vi "AlazarSetClockSwitchOver.vi"(3 "error in (no error)":errorcluster, 4 "DummyClockOnTime_ns":u32, 5 "Mode":u32(ring) items=["Disable", "Enable"], 6 "Handle":u64) -> (0 "error out":errorcluster, 1 "Return Code":u32, 2 "Handle":u64)   [LabVIEW 2009]
doc: "Configure the dummy clock.\n\nWhen the \"dummy clock\" option enabled, the digitizer uses an internally generated clock signal to drive its ADCs for a specified amount of time after the end of each record. At the end of the dummy clock on time, the digitizer switches back to using the external clock signal to clock the ADCs.\n\nScanning applications that generate an unusable external clock signal during horizontal retrace periods at the end of each scan line should consider enabling the \"dummy clock\" option."
uses:
  ATSApi.dll
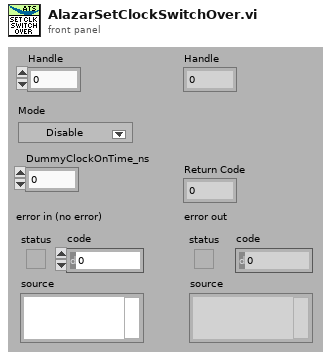
[diagram p1: front panel]
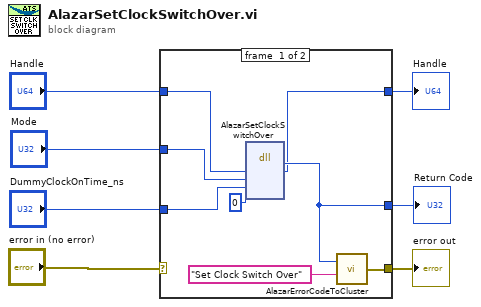
[diagram p0: block diagram]
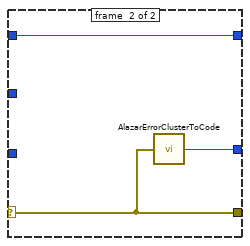
[diagram p2: hidden frame]
diagram:
  n1 = case shown="No Error" "error in (no error)" {
    selector: "error in (no error)" -> [_ w18]
    tunnel: [w12 w18] -> w6
    tunnel: [w14 w17] -> w5
    tunnel: "Handle" -> [w15 w16]
    tunnel: [w11 w16] -> w3
    tunnel: "Mode" -> [w10 _]
    tunnel: "DummyClockOnTime_ns" -> [w9 _]
    frame #0 {
      n2 = dll-call lib="ATSApi.dll" fn="AlazarSetClockSwitchOver"("handle"=w15, "mode"=w10, "dummyClockOnTime_ns"=w9, "reserved"=u32 0) -> ("return type"=w14:u32, "handle"=w11:u64)  [unwired: 6 in, 2 out]
      n3 = call "AlazarErrorCodeToCluster.vi"("Message"="Set Clock Switch Over", "Error Code"=w14) -> ("error out"=w12:errorcluster)
    }
    frame #1 {
      n4 = call "AlazarErrorClusterToCode.vi"("error in (no error)"=w18) -> ("Error Code"=w17:u32)
    }
  }
  "Handle" <- w3
  "error out" <- w6
  "Return Code" <- w5
